vi "Logarithm Fit (LAR).vi"(0 "Y":dbl[](array[numeric]), 5 "X":dbl[](array[numeric]), 7 "Weight":dbl[](array[numeric]), 9 "base of logarithm":dbl(ring)=2.71828 items=["e"=2.71828, "2"=2.0, "10"=10.0], 11 "tol":dbl=-1.0) -> (4 "Best Logarithm Fit":dbl[](array[numeric]), 6 "amplitude":dbl, 8 "scale":dbl, 14 "residue":dbl, 15 "error":i32)   [LabVIEW 2017, in "NI_AALPro.lvlib"]
uses:
  NI_AALPro.lvlib
  <resource>/lvanlys.dll
panel:
  # "LAR Logarithm Fit"
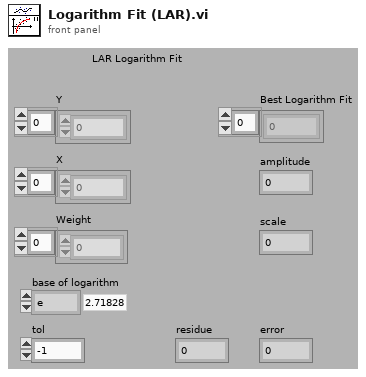
[diagram p1: front panel]
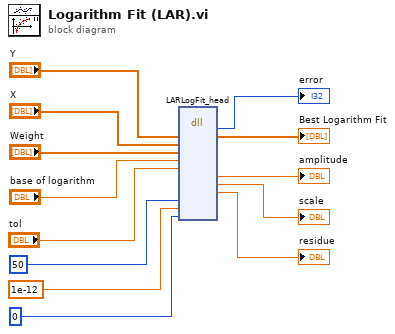
[diagram p0: block diagram]
diagram:
  n1 = dll-call lib="C:/Program Files (x86)/National Instruments/LabVIEW 2017/resource/lvanlys.*" fn="LARLogFit_head"("yH"="Y", "xH"="X", "weight"="Weight", "base"="base of logarithm", "tol"="tol", "maxIter"=50, "absTol"=1e-12, "isCoef"=0) -> (→"error":i32, "yH"=→"Best Logarithm Fit":dbl[], "amplitude"=→"amplitude":dbl, "scale"=→"scale":dbl, "meanErr"=→"residue":dbl)  [unwired: 13 in, 2 out]
